vi "CoMP-S Mechanism - Focus Verification.vi"(8 "error in (no error)":errorcluster, 10 "Motors":bool, 11 "Focus":T1=70.0 min=15.0 max=155.0 format="%.2f") -> (0 "error out":errorcluster, 3 "Focus out":dbl format="%#.1f")   [LabVIEW 2014]
uses:
  Controls/focus.ctl
panel:
  out "String 2":string
  in  "OK":bool
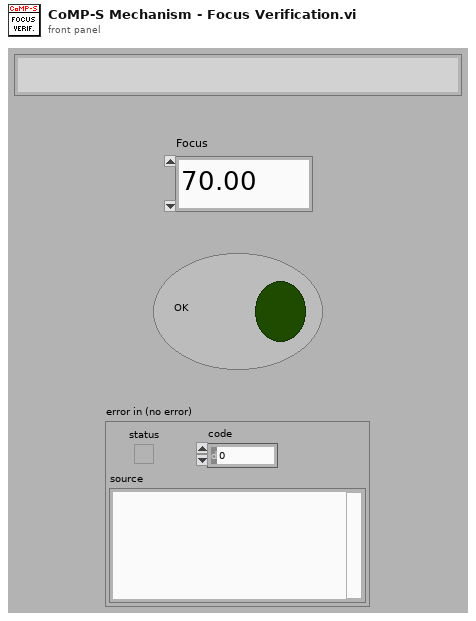
[diagram p1: front panel]
types:
  T1 = typedef "focus.ctl" = dbl
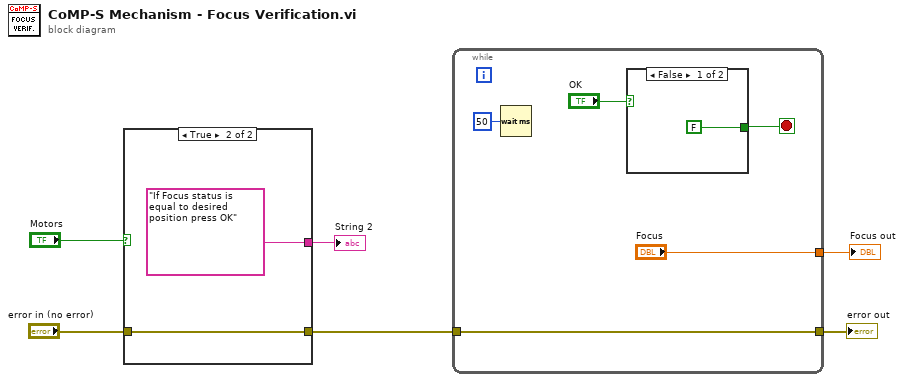
[diagram p0: block diagram]
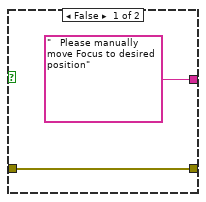
[diagram p2: hidden frame]
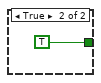
[diagram p3: hidden frame]
diagram:
  n1 = case shown="True" "Motors" {
    tunnel: ["   Please manually move Focus to desired position" ("String") "If Focus status is equal to desired position press OK" ("String")] -> w4
    tunnel: [w8 w9] -> w5
    tunnel: "error in (no error)" -> [w8 w9]
    frame False {
    }
    frame True {
    }
  }
  "String 2" <- w4
  n2 = while {
    tunnel: w5 -> [w12]
    tunnel: [w12] -> w6
    tunnel: ["Focus"] -> w1
    stop <- w13 stop-if-true
    n3 = Wait (ms)(milliseconds to wait=u32 50) -> ()  [unwired: 1 out]
    n4 = case shown="False" "OK" {
      tunnel: [FALSE TRUE] -> w13
      frame False {
      }
      frame True {
      }
    }
  }
  "error out" <- w6
  "Focus out" <- w1
